vi "EXTREME 3D Logitech Joystick Layout 6740.vi"(11 "Joystick Name":string="My Joystick RefNum") -> (0 "Logitech Joystick Buttons":T1, 3 "Logitech Joystick Axis":T2, 4 "POVs":i16[](array[numeric]))   [LabVIEW 2020]
uses:
  <vilib>/Rock Robotics/WPI/Utilities/WPI_GetSetVariantRefNum.vi
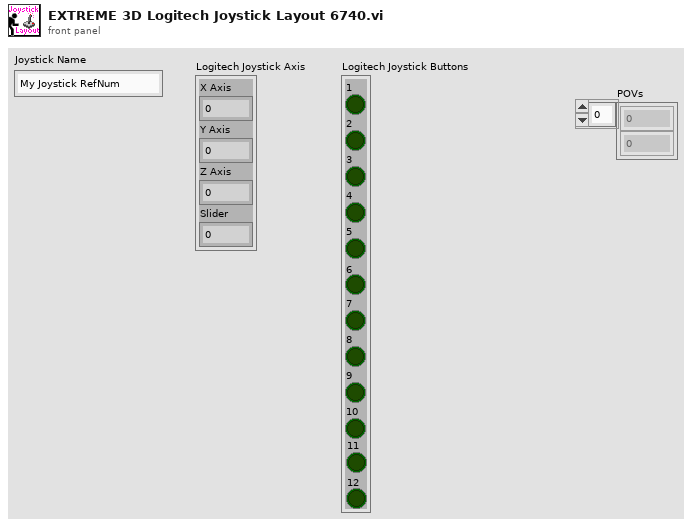
[diagram p1: front panel]
types:
  T1 = cluster{"1":bool, "2":bool, "3":bool, "4":bool, "5":bool, "6":bool, "7":bool, "8":bool, "9":bool, "10":bool, "11":bool, "12":bool}
  T2 = cluster{"X Axis":dbl, "Y Axis":dbl, "Z Axis":dbl, "Slider":dbl}
  T3 = typedef "WPI_JoystickDevRef.ctl" = cluster{"Device":T4}
  T4 = typedef "WPI_JoystickDeviceEnum.ctl" = enum16{"USB 0", "USB 1", "USB 2", "USB 3", "USB 4", "USB 5"}
  T5 = cluster{"Axes[0]":dbl, "Axes[1]":dbl, "Axes[2]":dbl, "Axes[3]":dbl, "Axes[4]":dbl, "Axes[5]":dbl, "Axes[6]":dbl, "Axes[7]":dbl, "Axes[8]":dbl}
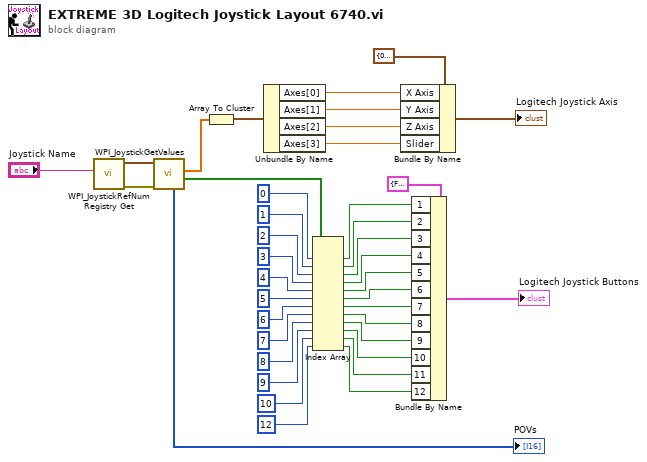
[diagram p0: block diagram]
diagram:
  n1 = call <vilib>:"WPI_JoystickRefNum Registry Get.vi"("refnum name"="Joystick Name") -> ("error out"=w28:errorcluster, "JoystickDevRef"=w30:T3)  [unwired: 9 in]
  n2 = call <vilib>:"WPI_JoystickGetValues.vi"("error in (no error)"=w28, "JoystickDevRef"=w30) -> ("Buttons"=w13:bool[], "Axes"=w15:dbl[], "POVs"=→"POVs":i16[])  [unwired: 5 in, 2 out]
  n3 = Array To Cluster(array=w15) -> (cluster=w14:T5)
  n4 = Unbundle By Name(w14) -> ("Axes[0]"=w38:dbl, "Axes[1]"=w37:dbl, "Axes[2]"=w36:dbl, "Axes[3]"=w35:dbl)
  n5 = Index Array(array=w13, index #1=0 ("index"), index #2=1 ("index"), index #3=2 ("index"), index #4=3 ("index"), index #5=4 ("index"), index #6=5 ("index"), index #7=6 ("index"), index #8=7 ("index"), index #9=8 ("index"), index #10=9 ("index"), index #11=10 ("index"), index #12=12 ("index")) -> (element #1=w12:bool, element #2=w11:bool, element #3=w10:bool, element #4=w9:bool, element #5=w8:bool, element #6=w7:bool, element #7=w6:bool, element #8=w5:bool, element #9=w4:bool, element #10=w3:bool, element #11=w2:bool, element #12=w1:bool)
  n6 = Bundle By Name(cluster=T2 {"X Axis"=0.0, "Y Axis"=0.0, "Z Axis"=0.0, "Slider"=0.0} ("input cluster"), "X Axis"=w38, "Y Axis"=w37, "Z Axis"=w36, "Slider"=w35) -> (→"Logitech Joystick Axis":T2)
  n7 = Bundle By Name(cluster=T1 {"1"=FALSE, "2"=FALSE, "3"=FALSE, "4"=FALSE, "5"=FALSE, "6"=FALSE, "7"=FALSE, "8"=FALSE, "9"=FALSE, "10"=FALSE, "11"=FALSE, "12"=FALSE} ("input cluster"), "1"=w12, "2"=w11, "3"=w10, "4"=w9, "5"=w8, "6"=w7, "7"=w6, "8"=w5, "9"=w4, "10"=w3, "11"=w2, "12"=w1) -> (→"Logitech Joystick Buttons":T1)
